vi "读取版本号.vi"() -> ()   [LabVIEW 2020]
uses:
  Global_Variable/Global.vi
  Libraries/ZLG_CAN/ZLG_CAN.lvlib
panel:
  in  "产品型号":u16(ring) items=["R92A", "R527", "R538"]
  out "硬件版本":string
  out "软件版本":string
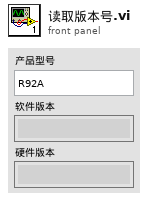
[diagram p1: front panel]
types:
  T1 = cluster{"波特率":u32, "ID":u32, "帧类型":enum8{"标准帧", "扩展帧"}, "帧格式":enum16{"数据帧", "远程帧"}, "周期(ms)":u32}
  T2 = cluster{"[0]":u8, "[1]":u8, "[2]":u8, "[3]":u8, "[4]":u8, "[5]":u8, "[6]":u8, "[7]":u8}[]
  T3 = typedef "ZLG_CAN.lvlib/Recive_Wait (Reply Payload)--cluster.ctl" = cluster{"Can_Receive":T4[], "Recive_Wait_error":errorcluster}
  T4 = typedef "ZLG_CAN.lvlib/CAN_OBJ_R.ctl" = cluster{"ID":u32, "TimeStamp":u32, "TimeFlag":u8, "SendType":u8, "RemoteFlag":u8, "ExternFlag":u8, "DataLen":u8, "数值":u8, "数值":u8, "数值":u8, "数值":u8, "数值":u8, "数值":u8, "数值":u8, "数值":u8, "数值":u8, "数值":u8, "数值":u8}
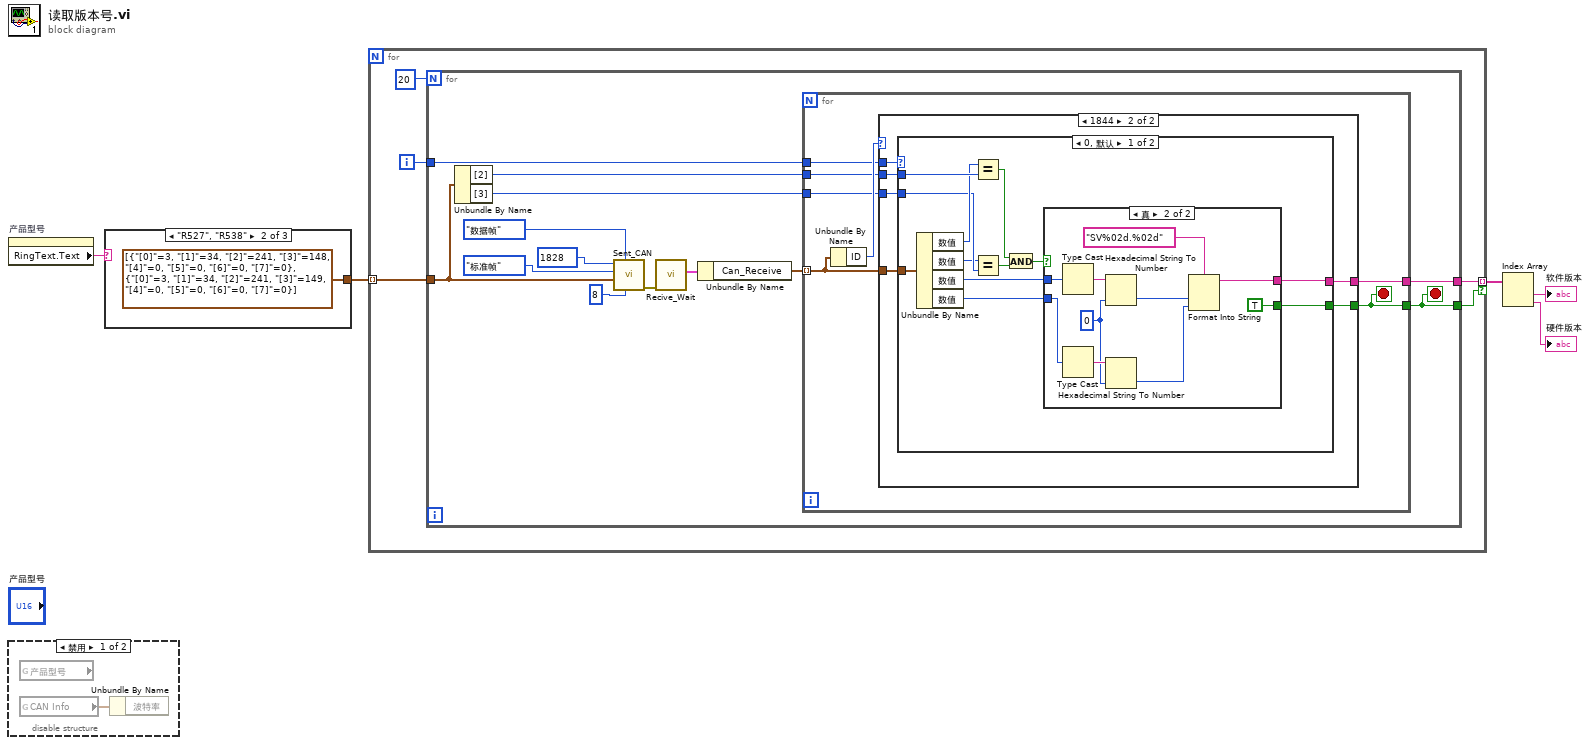
[diagram p0: block diagram]
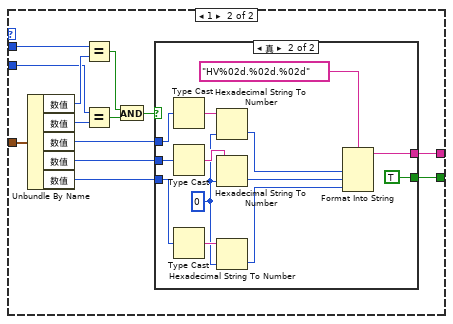
[diagram p5: hidden frame]
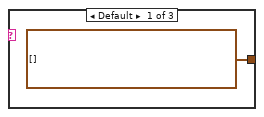
[diagram p7: hidden frame]
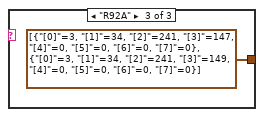
[diagram p8: hidden frame]
diagram:
  n1 = property on="产品型号" class="Ring (严格)"() -> ("RingText.Text"=w1:string)  [unwired: 2 in, 2 out]
  n2 = disable-structure shown="禁用" {
    frame Disabled {
      n3 = global read "Global.vi" "产品型号"() -> ()  [unwired: 1 out]
      n4 = global read "Global.vi" "CAN Info"() -> (w6:T1)
      n5 = Unbundle By Name(w6) -> ()  [unwired: 1 out]
    }
    frame Enabled {
    }
  }
  n6 = case shown="\"R527\", \"R538\"" w1 {
    tunnel: [T2 [] T2 [{"[0]"=3, "[1]"=34, "[2]"=241, "[3]"=148, "[4]"=0, "[5]"=0, "[6]"=0, "[7]"=0}, {"[0]"=3, "[1]"=34, "[2]"=241, "[3]"=149, "[4]"=0, "[5]"=0, "[6]"=0, "[7]"=0}] T2 [{"[0]"=3, "[1]"=34, "[2]"=241, "[3]"=147, "[4]"=0, "[5]"=0, "[6]"=0, "[7]"=0}, {"[0]"=3, "[1]"=34, "[2]"=241, "[3]"=149, "[4]"=0, "[5]"=0, "[6]"=0, "[7]"=0}]] -> w5
    frame Default {
    }
    frame "R527", "R538" {
    }
    frame "R92A" {
    }
  }
  n7 = for {
    tunnel: w5 -> [w14] mode=indexing
    tunnel: [w11] -> w4 mode=indexing if=w10
    i -> [w12]
    n8 = for {
      N: 20 -> [_]
      tunnel: w14 -> [w18]
      tunnel: w12 -> [w26]
      tunnel: [w25] -> w11
      tunnel: [w15] -> w10
      stop <- w15 stop-if-true
      n9 = Unbundle By Name(w18) -> ("[2]"=w17:u8, "[3]"=w16:u8)
      n10 = call "Sent_CAN.vi"("帧长度"=u8 8, "帧类型"=enum16{"数据帧", "远程帧"}."数据帧" ("帧格式"), "帧数据"=w18, "帧格式"=enum8{"标准帧", "扩展帧"}."标准帧" ("帧类型"), "ID"=u32 1828) -> ("error out"=w20:errorcluster)  [unwired: 6 in]
      n11 = call "Recive_Wait.vi"("error in (no error)"=w20) -> ("Reply Payload"=w19:T3)  [unwired: 8 in, 2 out]
      n12 = Unbundle By Name(w19) -> ("Can_Receive"=w27:T4[])
      n13 = for {
        tunnel: w27 -> [w33] mode=indexing
        tunnel: w26 -> [w32]
        tunnel: [w31] -> w25
        tunnel: w17 -> [w30]
        tunnel: w16 -> [w29]
        tunnel: [w28] -> w15
        stop <- w28 stop-if-true
        n14 = Unbundle By Name(w33) -> ("ID"=w34:u32)
        n15 = case shown="1844" w34 {
          tunnel: w33 -> [_ w40]
          tunnel: [_ w39] -> w31
          tunnel: [_ w35] -> w28
          tunnel: w32 -> [_ w38]
          tunnel: w30 -> [_ w37]
          tunnel: w29 -> [_ w36]
          frame 0, Default {
          }
          frame 1844 {
            n16 = case shown="0, 默认" w38 {
              tunnel: w40 -> [w52 w75]
              tunnel: [w49 w74] -> w39
              tunnel: w37 -> [w48 w67]
              tunnel: w36 -> [w46 w66]
              tunnel: [w41 w63] -> w35
              frame 0, Default {
                n17 = Unbundle By Name(w52) -> ("数值"=w47:u8, "数值"=w45:u8, "数值"=w51:u8, "数值"=w50:u8)
                n18 = Equal?(x=w47, y=w48) -> (x = y?=w44:bool)
                n19 = Equal?(x=w45, y=w46) -> (x = y?=w43:bool)
                n20 = And(x=w44, y=w43) -> (x .and. y?=w42:bool)
                n21 = case shown="真" w42 {
                  tunnel: w51 -> [_ w60]
                  tunnel: w50 -> [_ w59]
                  tunnel: [_ w55] -> w49
                  tunnel: [_ TRUE] -> w41
                  frame False {
                  }
                  frame True {
                    w54 = u8 0 ("默认(0 U32)")
                    n22 = Type Cast(x=w60) -> (*(type *) &x=w62:string)  [unwired: 1 in]
                    n23 = Type Cast(x=w59) -> (*(type *) &x=w61:string)  [unwired: 1 in]
                    n24 = Hexadecimal String To Number(string=w62, default (0uL)=w54) -> (number=w57:u8)  [unwired: 1 in, 1 out]
                    n25 = Hexadecimal String To Number(string=w61, default (0uL)=w54) -> (number=w56:u8)  [unwired: 1 in, 1 out]
                    n26 = Format Into String(format string="SV%02d.%02d" ("格式字符串"), w57, w56) -> (resulting string=w55:string)  [unwired: 2 in, 1 out]
                  }
                }
              }
              frame 1 {
                n27 = Unbundle By Name(w75) -> ("数值"=w68:u8, "数值"=w65:u8, "数值"=w73:u8, "数值"=w72:u8, "数值"=w71:u8)
                n28 = Equal?(x=w67, y=w68) -> (x = y?=w70:bool)
                n29 = Equal?(x=w66, y=w65) -> (x = y?=w69:bool)
                n30 = And(x=w70, y=w69) -> (x .and. y?=w64:bool)
                n31 = case shown="真" w64 {
                  tunnel: [_ w80] -> w74
                  tunnel: w73 -> [_ w79]
                  tunnel: w72 -> [_ w78]
                  tunnel: w71 -> [_ w77]
                  tunnel: [_ TRUE] -> w63
                  frame False {
                  }
                  frame True {
                    w82 = u8 0 ("默认(0 U32)")
                    n32 = Type Cast(x=w79) -> (*(type *) &x=w86:string)  [unwired: 1 in]
                    n33 = Type Cast(x=w78) -> (*(type *) &x=w85:string)  [unwired: 1 in]
                    n34 = Type Cast(x=w77) -> (*(type *) &x=w87:string)  [unwired: 1 in]
                    n35 = Hexadecimal String To Number(string=w86, default (0uL)=w82) -> (number=w84:u8)  [unwired: 1 in, 1 out]
                    n36 = Hexadecimal String To Number(string=w85, default (0uL)=w82) -> (number=w83:u8)  [unwired: 1 in, 1 out]
                    n37 = Hexadecimal String To Number(string=w87, default (0uL)=w82) -> (number=w88:u8)  [unwired: 1 in, 1 out]
                    n38 = Format Into String(format string="HV%02d.%02d.%02d" ("格式字符串"), w84, w83, w88) -> (resulting string=w80:string)  [unwired: 2 in, 1 out]
                  }
                }
              }
            }
          }
        }
      }
    }
  }
  n39 = Index Array(array=w4) -> (element #1=→"软件版本":string, element #2=→"硬件版本":string)  [unwired: 2 in]
